vi "decodeBin.vi"(8 "error in (no error)":errorcluster, 10 "ByteArray":u8[](array[numeric])) -> (0 "error out":errorcluster, 1 "BinaryArray":u8[](array[numeric]), 2 "variant":variant, 3 "RemainingBytes":u8[](array[numeric]), 5 "Type":string)   [LabVIEW 2020, in "MsgPack.lvlib"]
uses:
  MsgPack.lvlib
  <vilib>/Utility/error.llb/Error Cluster From Error Code.vi
  <vilib>/ErrorRing/Error Ring.xnode
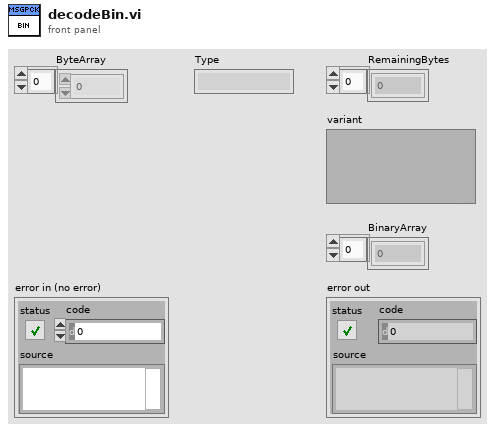
[diagram p1: front panel]
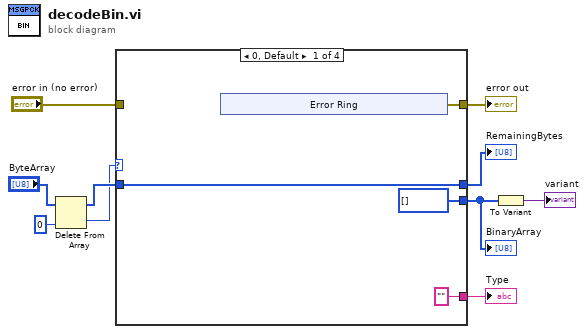
[diagram p0: block diagram]
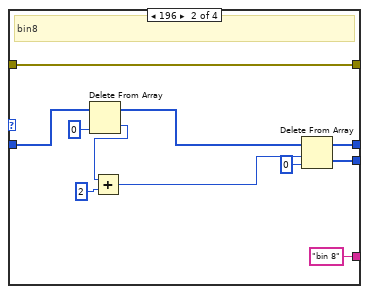
[diagram p2: hidden frame]
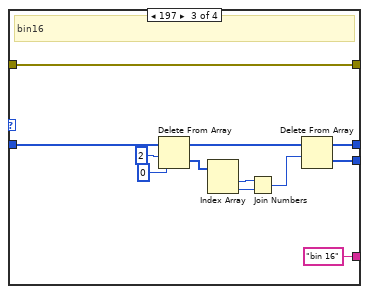
[diagram p3: hidden frame]
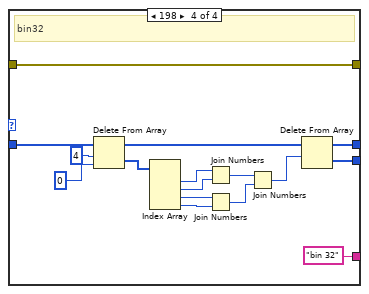
[diagram p4: hidden frame]
diagram:
  n1 = Delete From Array(array="ByteArray", index=0) -> (deleted portion=w1:u8, array with subset deleted=w3:u8[])  [unwired: 1 in]
  n2 = case shown="0, Default" w1 {
    tunnel: [w13 w28 w41 w57] -> w9
    tunnel: "error in (no error)" -> [_ w28 w41 w57]
    tunnel: ["" "bin 8" "bin 16" "bin 32"] -> w7
    tunnel: [u8[] [] w25 w33 w45] -> w6
    tunnel: w3 -> [w11 w22 w36 w50]
    tunnel: [w11 w26 w32 w44] -> w5
    frame 0, Default {
      n3 = xnode "Error Ring"() -> ("error out"=w13:errorcluster)
    }
    frame 196 {
      # "bin8"
      n4 = Delete From Array(array=w22, index=0) -> (deleted portion=w21:u8, array with subset deleted=w20:u8[])  [unwired: 1 in]
      n5 = Add(x=w21, y=u8 2) -> (x+y=w27:u8)
      n6 = Delete From Array(array=w20, length=w27, index=0) -> (deleted portion=w25:u8[], array with subset deleted=w26:u8[])
    }
    frame 197 {
      # "bin16"
      n7 = Delete From Array(array=w36, length=2, index=0) -> (deleted portion=w37:u8[], array with subset deleted=w35:u8[])
      n8 = Index Array(array=w37) -> (element #1=w39:u8, element #2=w40:u8)  [unwired: 2 in]
      n9 = Join Numbers(hi=w39, lo=w40) -> ((hi.lo)=w34:u16)
      n10 = Delete From Array(array=w35, length=w34) -> (deleted portion=w33:u8[], array with subset deleted=w32:u8[])  [unwired: 1 in]
    }
    frame 198 {
      # "bin32"
      n11 = Delete From Array(array=w50, length=4, index=0) -> (deleted portion=w48:u8[], array with subset deleted=w47:u8[])
      n12 = Index Array(array=w48) -> (element #1=w55:u8, element #2=w56:u8, element #3=w54:u8, element #4=w53:u8)  [unwired: 4 in]
      n13 = Join Numbers(hi=w55, lo=w56) -> ((hi.lo)=w51:u16)
      n14 = Join Numbers(hi=w54, lo=w53) -> ((hi.lo)=w52:u16)
      n15 = Join Numbers(hi=w51, lo=w52) -> ((hi.lo)=w46:u32)
      n16 = Delete From Array(array=w47, length=w46) -> (deleted portion=w45:u8[], array with subset deleted=w44:u8[])  [unwired: 1 in]
    }
  }
  "error out" <- w9
  "Type" <- w7
  "BinaryArray" <- w6
  "RemainingBytes" <- w5
  n17 = To Variant(anything=w6) -> (Variant=→"variant":variant)
